vi "Update Clock.vi"(6 "timeout (ms)":i32=5000, 8 "error in":errorcluster, 10 "Clock Update":T1, 11 "gRPC ID in":T3) -> (0 "error out":errorcluster, 3 "gRPC ID out":T3)   [LabVIEW 2021, in "CIFManagerClientWrapper.lvlib"]
uses:
  CIFManagerClientWrapper.lvlib
  CIF_Manager_client/CIF_Manager_client.lvlib
  CIF_Manager_client/RPC Messages/cif_manager_TimePair.ctl
  CIF_Manager_client/RPC Messages/cif_manager_ClockUpdate.ctl
  <vilib>/gRPC/LabVIEW gRPC Library/Shared/grpcId.ctl
  <vilib>/gRPC/LabVIEW gRPC Library/grpc-lvsupport-release.lvlib
  <vilib>/CIF Foundation/CIF Utilities/Time/Typedef/Timestamp Pair.ctl
  <vilib>/CIF Foundation/CIF Utilities/Time/Time_CIF_U.lvlib
  <vilib>/CIF Foundation/CIF Utilities/Time/Typedef/Clock Update.ctl
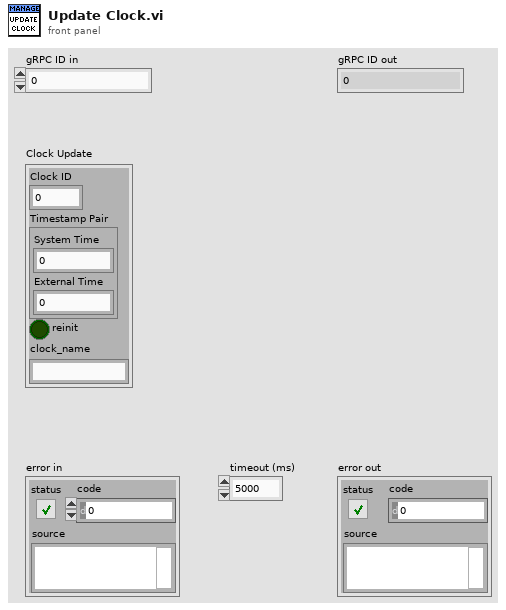
[diagram p1: front panel]
types:
  T1 = typedef "Time_CIF_U.lvlib/Clock Update.ctl" = cluster{"Clock ID":u8, "Timestamp Pair":T2, "reinit":bool, "clock_name":string}
  T2 = typedef "Time_CIF_U.lvlib/Timestamp Pair.ctl" = cluster{"System Time":i64, "External Time":i64}
  T3 = typedef "grpc-lvsupport-release.lvlib/grpcId.ctl" = u64
  T4 = typedef "CIF_Manager_client.lvlib/cif_manager_ClockUpdate.ctl" = cluster{"clock_id":u32, "timestamp_pair":T5, "reinit":bool, "clock_name":string}
  T5 = typedef "CIF_Manager_client.lvlib/cif_manager_TimePair.ctl" = cluster{"system_time":i64, "external_time":i64}
  T6 = typedef "CIF_Manager_client.lvlib/cif_manager_Error.ctl" = cluster{"message":string, "code":i32}
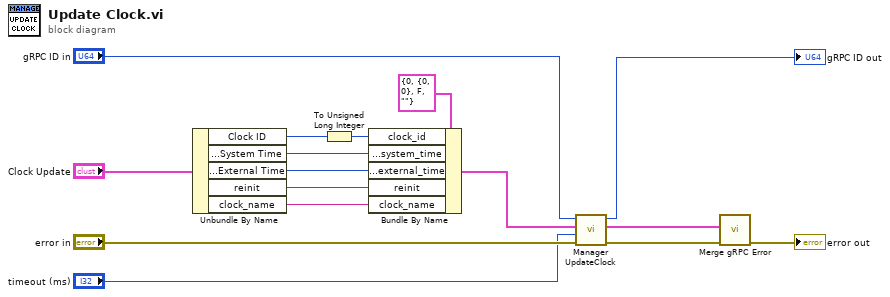
[diagram p0: block diagram]
diagram:
  n1 = Unbundle By Name("Clock Update") -> ("Clock ID"=w6:u8, "Timestamp Pair.System Time"=w2:i64, "Timestamp Pair.External Time"=w3:i64, "reinit"=w4:bool, "clock_name"=w5:string)
  n2 = To Unsigned Long Integer(number=w6) -> (unsigned 32bit integer=w1:u32)
  n3 = Bundle By Name(cluster=T4 {"clock_id"=0, "timestamp_pair"={"system_time"=0, "external_time"=0}, "reinit"=FALSE, "clock_name"=""} ("Request Data"), "clock_id"=w1, "timestamp_pair.system_time"=w2, "timestamp_pair.external_time"=w3, "reinit"=w4, "clock_name"=w5) -> (w7:T4)
  n4 = call "Manager UpdateClock.vi"("error in"="error in", "timeout (ms)"="timeout (ms)", "Request Data"=w7, "gRPC ID"="gRPC ID in") -> ("error out"=w11:errorcluster, "Response Data"=w12:T6, "gRPC ID out"=→"gRPC ID out":T3)  [unwired: 5 in]
  n5 = call "Merge gRPC Error.vi"("error in (no error)"=w11, "gRPC Error"=w12) -> ("error out"=→"error out":errorcluster)  [unwired: 9 in]
